vi "LabVIEW2018_RS232_loopback_test.vi"() -> ()   [LabVIEW 2019]
uses:
  <vilib>/Instr/_visa.llb/VISA Configure Serial Port (Instr).vi
panel:
  in  "Delay Time (s)":dbl=0.5 format="%#_13g"
  in  "Send":bool
  in  "Flow control":u16(ring) items=["None", "XON/XOFF", "RTS/CTS", "XON/XOFF & RTS/CTS", "DTR/DSR", "XON/XOFF & DTR/DSR"]
  in  "Stop bits":u16(ring)=10 items=["1.0"=10, "1.5"=15, "2.0"=20]
  in  "Parity":enum16{"None", "Odd", "Even", "Mark", "Space"}(ring)
  in  "Data bits":u16=8
  in  "Baud rate":u32=9600
  in  "Sent Message":string="meas1?"
  in  "VISA resource name":refnum<visa-resource-name>="COM3"
  out "Read Response":string
  in  "stop":bool
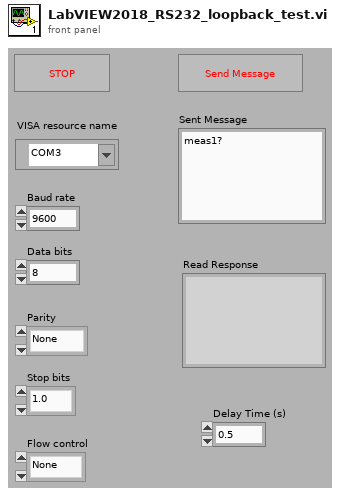
[diagram p1: front panel]
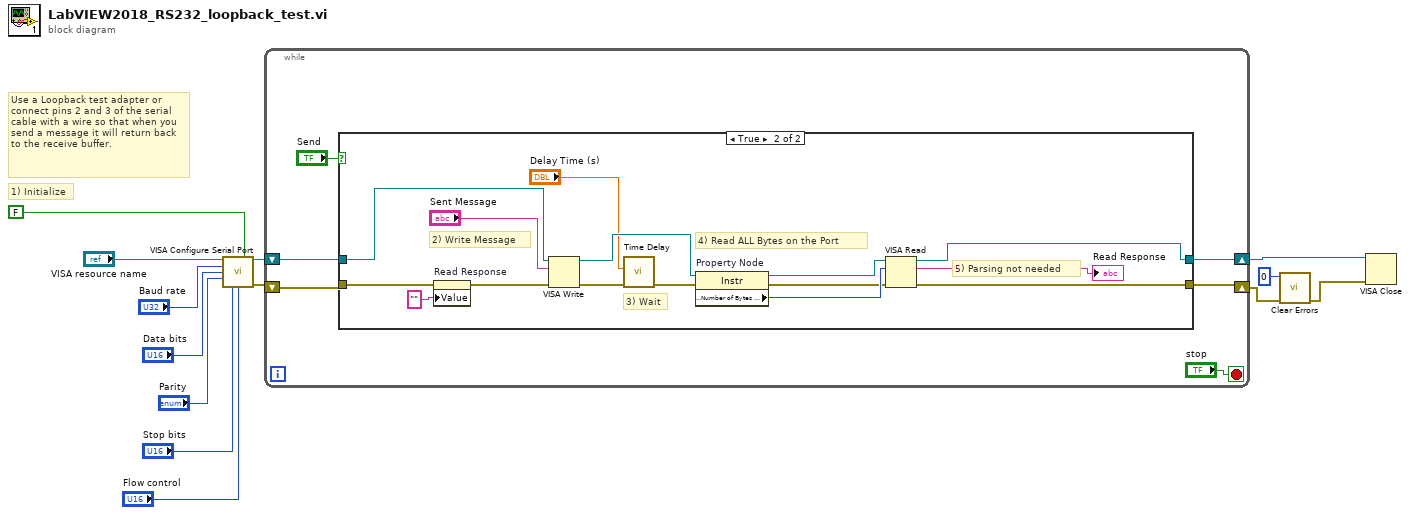
[diagram p0: block diagram]
diagram:
  # "Use a Loopback test adapter or connect pins 2 and 3 of the serial cable with a wire so that when you send a message it will return back to the receive buffer."
  # "1) Initialize"
  n1 = call-poly "VISA Configure Serial Port"("VISA resource name"="VISA resource name", "Enable Termination\nChar (T)"=FALSE ("Enable Termination\nChar (T)"), "baud rate (9600)"="Baud rate", "data bits (8)"="Data bits", "parity (0:none)"="Parity", "stop bits (10: 1 bit)"="Stop bits", "flow control (0:none)"="Flow control") -> ("VISA resource name out"=w7:refnum<visa-resource-name>, "error out"=w6:errorcluster)  [unwired: 1 in, 6 out]
  n2 = while {
    shift-right: [w16] -> w5
    shift-left: w7 -> [w19]
    shift-right: [w15] -> w4
    shift-left: w6 -> [w18]
    stop <- "stop" stop-if-true
    n3 = case shown="True" "Send" {
      tunnel: w19 -> [w21 w36]
      tunnel: w18 -> [w20 w23]
      tunnel: [w21 w35] -> w16
      tunnel: [w20 w34] -> w15
      frame False {
      }
      frame True {
        # "5) Parsing not needed"
        # "3) Wait"
        # "2) Write Message"
        # "4) Read ALL Bytes on the Port"
        n4 = property on="Read Response" class="Str"(error in=w23, "Value"="" ("Read Response")) -> (error out=w22:errorcluster)  [unwired: 1 in, 1 out]
        n5 = VISA Write(VISA resource name=w36, write buffer="Sent Message", error in (no error)=w22) -> (VISA resource name out=w28:refnum<visa-resource-name>, error out=w30:errorcluster)  [unwired: 1 out]
        n6 = call "Time Delay"("error in (no error)"=w30, "Delay Time (s)"="Delay Time (s)") -> ("error out"=w29:errorcluster)  [unwired: 9 out]
        n7 = property on="Property Node" class="Instr"(reference=w28, error in=w29) -> (reference out=w32:refnum<visa-resource-name>, error out=w31:errorcluster, "Serial Settings:Number of Bytes at Serial Port"=w33:u32)
        n8 = VISA Read(VISA resource name=w32, byte count=w33, error in (no error)=w31) -> (VISA resource name out=w35:refnum<visa-resource-name>, read buffer=→"Read Response":string, error out=w34:errorcluster)  [unwired: 1 out]
      }
    }
  }
  n9 = call <vilib>:"Clear Errors.vi"("error in (no error)"=w4, "specific error code to clear (0: all)"=0) -> ("error out"=w2:errorcluster)  [unwired: 4 in, 1 out]
  n10 = VISA Close(VISA resource name=w5, error in (no error)=w2) -> ()  [unwired: 1 out]
